vi "FSK.vi"() -> ()   [LabVIEW 2009]
uses:
  <vilib>/addons/Modulation/Analog/MT Downconvert Passband (Real).vi
  <vilib>/addons/Modulation/Analog/MT Upconvert Baseband (Real).vi
  <vilib>/addons/Modulation/Digital/General/MT Generate Bits (Galois, PN Order).vi
  <vilib>/Analysis/4window.llb/windowTd.ctl
  <vilib>/measure/maspectr.llb/FFT Power Spectrum for 1 Chan.vi
  Instance          11 16Saved   FSK-rev2 .vi
  <vilib>/Analysis/NI_AALPro.lvlib
  <vilib>/measure/NI_MAPro.lvlib
panel:
  in  "Tab Control":enum32{"Time Domain", "Frequency Domain"}(tab)
  out "Passband time domain signal":waveform(dbl)[](graph)=[{"t0"=timestamp(0 s since 1904-01-01), "dt"=4.166666666666667e-11, "Y"=array[25601 elements]}]
  out "Power Spectrum":cluster{"f0":dbl, "df":dbl, "spectrum":dbl[]}(graph)={"f0"=0.0, "df"=933815.8048324967, "spectrum"=array[12851 elements]}
  in  "symbol phase continuity":enum16{"continuous", "discontinuous"}(ring)=enum."discontinuous"
  out "df":dbl=933815.8048324967 format="%#_6p"
  in  "Frequency Deviation from Carrier (+/-)":dbl=500000000.0 format="%#_6p"
  in  "Random Sequence / 1010 Sequence":bool
  in  "modulation type 2":enum16{"FSK", "PSK", "QAM", "MSK", "PAM", "ASK"}(ring)
  in  "Delay per cycle (Seconds)":dbl=1.0 caption="Delay Time (s)"
  out "Symbol Period":dbl=8.333333333333334e-09
  out "Number of Bit Errors":i8
  out "Decoded Bits (16 shown at a time, scroll to view remainder)":i8[](array[numeric])=[0, 0, 0, 0, 1, 0, 0, 0, 0, 1, 1, 0, 0, 0, 1, 0, 1, 0, 0, 1, 1, 1, 1, 0, 1, 0, 0, 0, 1, 1, 1, 0, 0, 1, 0, 0, 1, 0, 1, 1, 0, 1, 1, 1, 0, 1, 1, 0, 0, 1, 1, 0, 1, 0, 1, 0, 1, 1, 1, 1, 1, 1, 0, 0, 0, 0, 0, 1, 0, 0, 0, 0, 1, 1, 0, 0, 0, 1, 0, 1, 0, 0, 1, 1, 1, 1, 0, 1, 0, 0, 0, 1, 1, 1, 0, 0, 1, 0, 0, 1, 0, 1, 1, 0, 1, 1, 1, 0, 1, 1, 0, 0, 1, 1, 0, 1, 0, 1, 0, 1, 1, 1, 1, 1, 1, 0]
  out "Signal Bandwidth":dbl=40000000.0 format="%#.6p"
  in  "Filter parameter (Rolloff Factor)":dbl=1.0 format="%.2f"
  in  "Carrier Frequency (Hz)":dbl=2000000000.0 min=-0.5 max=0.5 format="%#.6p"
  in  "modulation type":enum16{"FSK", "PSK", "QAM", "MSK", "PAM", "ASK"}(ring)=enum."ASK"
  in  "pulse shaping filter (none)":T1(ring)
  in  "filter length (symbols)":i32=8
  in  "Symbol Rate (Hz)":dbl=10000000.0 format="%#.6p"
  in  "Terminate Simulation":bool
  out "Bits (16 shown at a time, scroll to view remainder of stream)":i8[](array[numeric])=[0, 0, 0, 0, 1, 0, 0, 0, 0, 1, 1, 0, 0, 0, 1, 0, 1, 0, 0, 1, 1, 1, 1, 0, 1, 0, 0, 0, 1, 1, 1, 0, 0, 1, 0, 0, 1, 0, 1, 1, 0, 1, 1, 1, 0, 1, 1, 0, 0, 1, 1, 0, 1, 0, 1, 0, 1, 1, 1, 1, 1, 1, 0, 0, 0, 0, 0, 1, 0, 0, 0, 0, 1, 1, 0, 0, 0, 1, 0, 1, 0, 0, 1, 1, 1, 1, 0, 1, 0, 0, 0, 1, 1, 1, 0, 0, 1, 0, 0, 1, 0, 1, 1, 0, 1, 1, 1, 0, 1, 1, 0, 0, 1, 1, 0, 1, 0, 1, 0, 1, 1, 1, 1, 1, 1, 0, 0, 0]
  in  "PN sequence order (Valid range 6-15)":i32=6 min=5 max=31
  in  "Number of Bits to Generate":i32=128
  in  "Bit Sequence Generation Type  (Galois PN, Uniform Random)":bool
  # "Configuration"
  # "(delayed due to group delay of passband / pulse shaping / etc filters)"
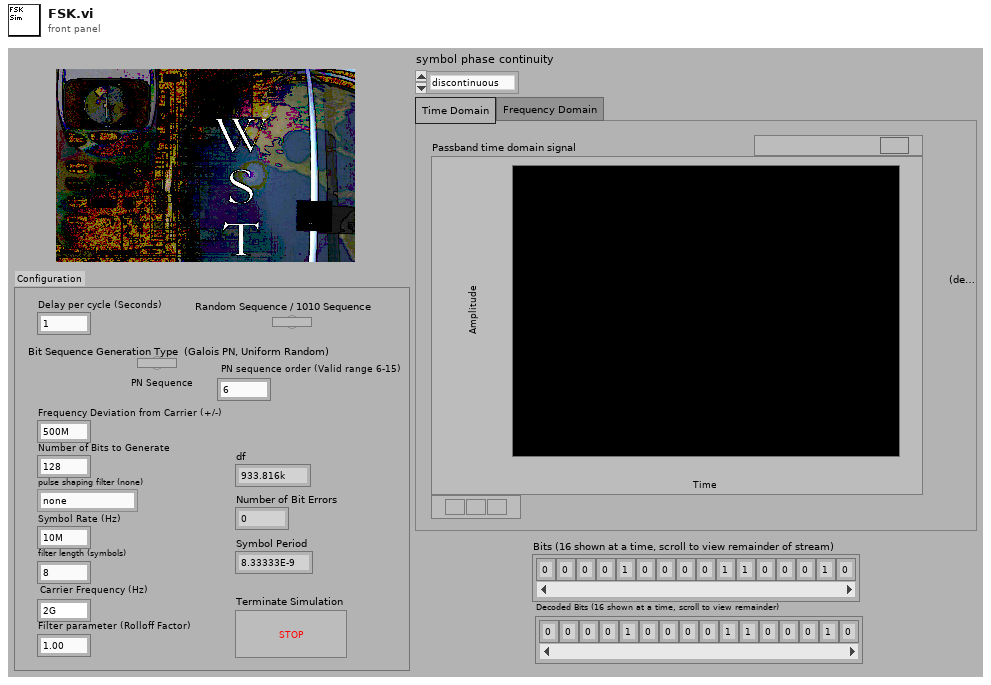
[diagram p1: front panel]
types:
  T1 = enum16{"none", "Raised Cosine", "Root Raised Cos"}
  T2 = enum16{"none", "Raised Cosine", "Root Raised Cos", "Gaussian"}
  T3 = cluster{"samples per symbol (16)":i32, "symbol map":dbl[], "symbol phase continuity":enum16{"continuous", "discontinuous"}}
  T4 = typedef "Complex Data Waveform.ctl" = cluster{"t0":dbl, "dt":dbl, "Y":cdb[]}
  T5 = typedef "NI_AALPro.lvlib/windowTd.ctl" = u32
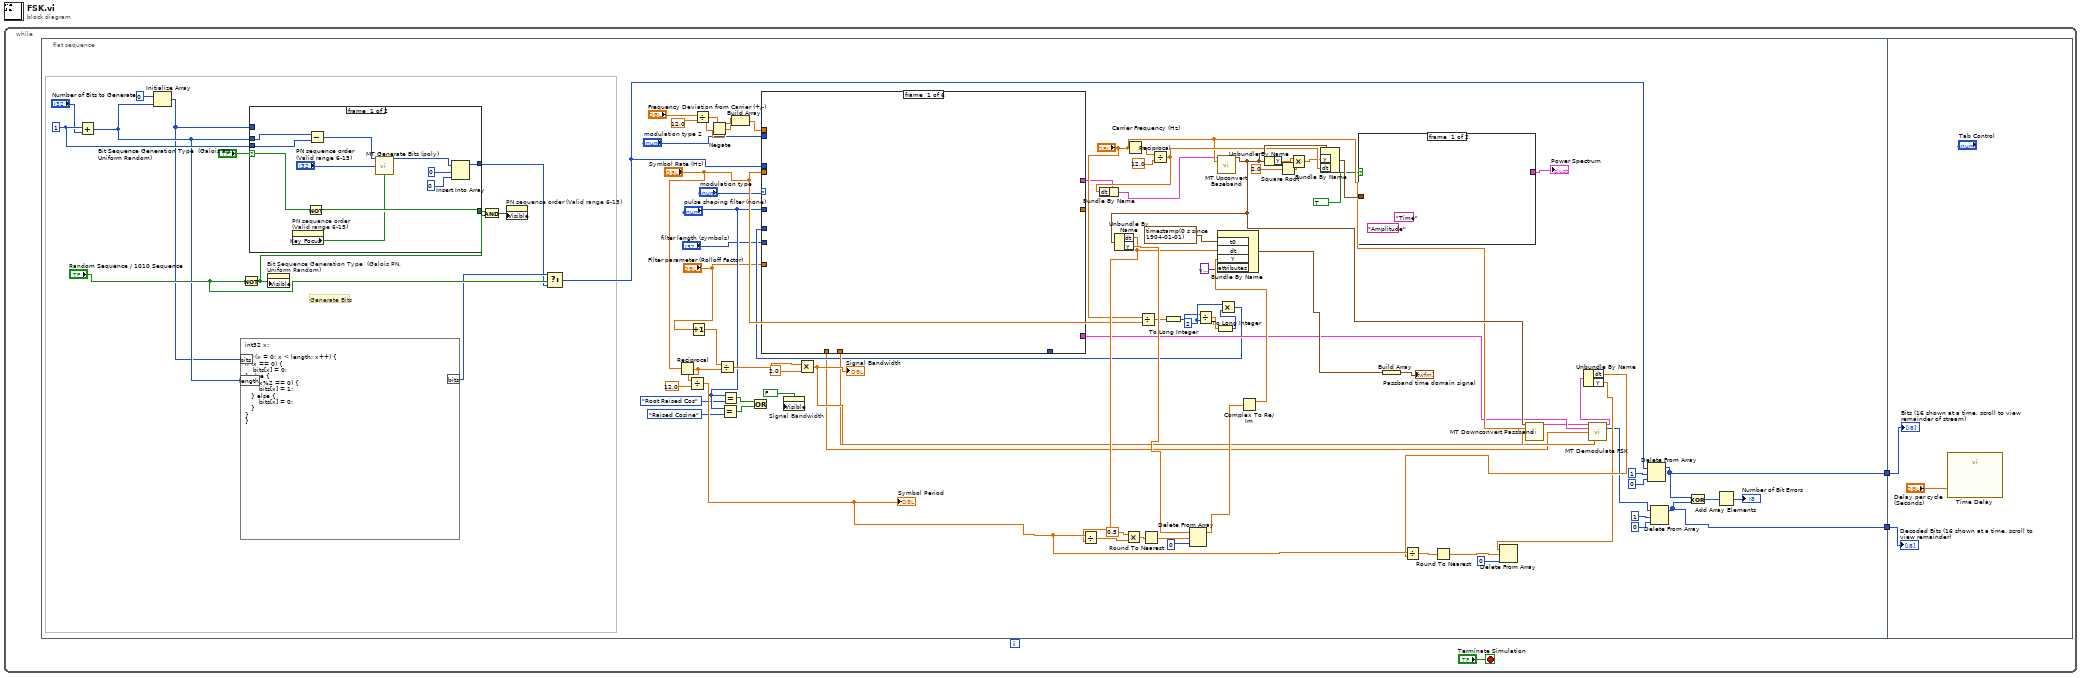
[diagram p0: block diagram]
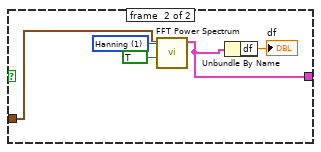
[diagram p2: hidden frame]
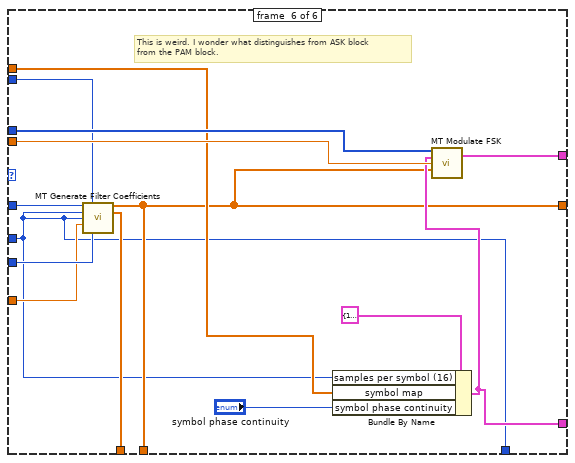
[diagram p7: hidden frame]
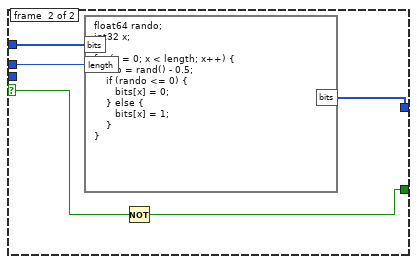
[diagram p8: hidden frame]
diagram:
  n1 = while {
    stop <- "Terminate Simulation" stop-if-true
    n2 = flat-sequence {
      tunnel: [w5] -> w2
      tunnel: [w4] -> w1
      tunnel: w2 -> [w128]
      tunnel: w1 -> [w127]
      frame #0 {
        w76 = 1 ("x")
        w21 = 2 ("y")
        # "Generate Bits"
        n3 = Add(x=w76, y="Number of Bits to Generate") -> (x+y=w50:i32)
        n4 = Initialize Array(i8 0, w50) -> (w49:i8[])
        n5 = formula code="int32 x;\n\nfor (x = 0; x < length; x++) {\nif (x == 0) {\n    bits[x] = 0;\n} else {\n   if (x%2 == 0) {\n       bits[x] = 1;\n   } else {\n       bits[x] = 0;\n   }\n}\n}"("bits"=w49, "length"=w50) -> ("bits"=w53:i8[])
        n6 = Not(x="Random Sequence / 1010 Sequence") -> (.not. x?=w57:bool)
        n7 = case shown="False" "Bit Sequence Generation Type  (Galois PN, Uniform Random)" {
          selector: "Bit Sequence Generation Type  (Galois PN, Uniform Random)" -> [w120 w123]
          tunnel: w50 -> [w113 w125]
          tunnel: [w114 w124] -> w52
          tunnel: w49 -> [_ w126]
          tunnel: [w119 w122] -> w55
          tunnel: w76 -> [w112 _]
          frame #0 {
            n8 = property on="PN sequence order (Valid range 6-15)" class="DigNum (strict)"() -> ("Key Focus"=w118:bool)  [unwired: 2 in, 2 out]
            n9 = Not(x=w120) -> (.not. x?=w119:bool)
            n10 = Subtract(x=w113, y=w112) -> (x-y=w117:i32)
            n11 = call-poly <vilib>:"MT Generate Bits (poly).vi"("total bits (128)"=w117, "PN sequence order (9)"="PN sequence order (Valid range 6-15)", "reset? (T)"=w118) -> ("output bit stream"=w115:i8[])  [unwired: 10 in, 2 out]
            n12 = Insert Into Array(array=w115, index=0, new element=i8 0 ("new element/subarray")) -> (w114:i8[])
          }
          frame #1 {
            n13 = formula code="float64 rando;\nint32 x;\n\nfor (x = 0; x < length; x++) {\nrando = rand() - 0.5;\n    if (rando <= 0) {\n       bits[x] = 0;\n    } else {\n       bits[x] = 1;\n    }\n}"("bits"=w126, "length"=w125) -> ("bits"=w124:i8[])
            n14 = Not(x=w123) -> (.not. x?=w122:bool)
          }
        }
        n15 = property on="Bit Sequence Generation Type  (Galois PN, Uniform Random)" class="Bool (strict)"("Visible"=w57) -> ()  [unwired: 2 in, 2 out]
        n16 = And(x=w55, y=w57) -> (x .and. y?=w56:bool)
        n17 = property on="PN sequence order (Valid range 6-15)" class="DigNum (strict)"("Visible"=w56) -> ()  [unwired: 2 in, 2 out]
        n18 = Select(t=w53, s="Random Sequence / 1010 Sequence", f=w52) -> (s? t:f=w85:i8[])
        n19 = Reciprocal(x="Symbol Rate (Hz)") -> (1/x=w30:dbl)
        n20 = Divide(x=w30, y=12.0) -> (x/y=w91:dbl)
        "Symbol Period" <- w91
        n21 = Increment(x="Filter parameter (Rolloff Factor)") -> (x+1=w11:dbl)
        n22 = Divide(x="Frequency Deviation from Carrier (+/-)", y=12.0) -> (x/y=w75:dbl)
        n23 = Negate(x=w75) -> (-x=w74:dbl)
        n24 = Divide(x=w11, y=w30) -> (x/y=w46:dbl)
        n25 = Equal?(x="pulse shaping filter (none)", y=T2."Raised Cosine") -> (x = y?=w13:bool)
        n26 = Equal?(x="pulse shaping filter (none)", y=T2."Root Raised Cos") -> (x = y?=w12:bool)
        n27 = Build Array(w74, w75) -> (w60:dbl[])
        n28 = Or(x=w12, y=w13) -> ()  [unwired: 1 out]
        n29 = property on="Signal Bandwidth" class="DigNum (strict)"("Visible"=FALSE) -> ()  [unwired: 2 in, 2 out]
        n30 = Multiply(x=w46, y=2.0) -> (x*y=w69:dbl)
        "Signal Bandwidth" <- w69
        n31 = Reciprocal(x="Carrier Frequency (Hz)") -> (1/x=w16:dbl)
        n32 = Divide(x="Carrier Frequency (Hz)", y="Symbol Rate (Hz)") -> (x/y=w19:dbl)
        n33 = Divide(x=w16, y=12.0) -> (x/y=w72:dbl)
        n34 = To Long Integer(number=w19) -> (32bit integer=w20:i32)
        n35 = Divide(x=w20, y=w21) -> (x/y=w22:dbl)
        n36 = To Long Integer(number=w22) -> (32bit integer=w23:i32)
        n37 = Multiply(x=w21, y=w23) -> (x*y=w26:i32)
        n38 = case shown="\"ASK\"" "modulation type" {
          tunnel: "Symbol Rate (Hz)" -> [_ _ _ _ _ w110]
          tunnel: "filter length (symbols)" -> [_ _ _ _ _ w109]
          tunnel: "pulse shaping filter (none)" -> [_ _ _ _ _ w108]
          tunnel: w85 -> [_ _ _ _ _ w107]
          tunnel: [_ _ _ _ _ w106] -> w61
          tunnel: "Filter parameter (Rolloff Factor)" -> [_ _ _ _ _ w105]
          tunnel: w26 -> [_ _ _ _ _ w97]
          tunnel: [_ _ _ _ _ w104] -> w25
          tunnel: "modulation type 2" -> [_ _ _ _ _ w103]
          tunnel: [_ _ _ _ _ w101] -> w58
          tunnel: [_ _ _ _ _ w98] -> w59
          tunnel: w60 -> [_ _ _ _ _ w100]
          tunnel: [_ _ _ _ _ w98] -> _
          tunnel: [_ _ _ _ _ w97] -> _
          frame #0 {
          }
          frame #1 {
          }
          frame #2 {
          }
          frame #3 {
          }
          frame #4 {
          }
          frame #5 {
            # "This is weird. I wonder what distinguishes from ASK block\nfrom the PAM block."
            n39 = call <vilib>:"MT Generate Filter Coefficients.vi"("pulse shaping filter (none)"=w108, "modulation type"=w103, "pulse shaping samples per symbol (16)"=w97, "matched samples per symbol (16)"=w97, "filter parameter"=w105, "filter length (symbols)"=w109) -> ("pulse shaping filter coefficients"=w98:dbl[], "matched filter coefficients"=w104:dbl[])  [unwired: 7 in, 1 out]
            n40 = Bundle By Name(cluster=T3 {"samples per symbol (16)"=16, "symbol map"=[], "symbol phase continuity"=enum."continuous"} ("FSK system parameters"), "samples per symbol (16)"=w97, "symbol map"=w100, "symbol phase continuity"="symbol phase continuity") -> (w101:T3)
            n41 = call <vilib>:"MT Modulate FSK.vi"("input bit stream"=w107, "FSK system parameters"=w101, "symbol rate (Hz)"=w110, "pulse shaping filter coefficients"=w98) -> ("output complex waveform"=w106:T4)  [unwired: 9 in, 2 out]
          }
        }
        n42 = Bundle By Name(cluster=w61, "dt"=w72) -> (w62:T4)
        n43 = call-poly <vilib>:"MT Upconvert Baseband.vi"("baseband waveform (complex)"=w62, "carrier frequency (Hz)"="Carrier Frequency (Hz)") -> ("passband waveform"=w87:waveform(dbl))  [unwired: 12 in, 1 out]
        n44 = Unbundle By Name(w87) -> ("dt"=w88:dbl, "Y"=w89:dbl[])
        n45 = Divide(x=w91, y=w88) -> (x/y=w77:dbl)
        n46 = Multiply(x=0.5, y=w77) -> (x*y=w79:dbl)
        n47 = Round To Nearest(number=w79) -> (nearest integer value=w90:dbl)
        n48 = Delete From Array(array=w89, length=w90, index=0) -> (array with subset deleted=w80:dbl[])  [unwired: 1 out]
        n49 = Complex To Re/Im(x + iy=w80) -> (x=w81:dbl[])  [unwired: 1 out]
        n50 = Bundle By Name("t0"=timestamp(0 s since 1904-01-01), "dt"=w88, "Y"=w81, "attributes"=variant) -> (w86:waveform(dbl))  [unwired: 1 in]
        n51 = Unbundle By Name(w87) -> ("Y"=w65:dbl[])
        n52 = Square Root(x=2.0) -> (sqrt(x)=w66:dbl)
        n53 = Multiply(x=w65, y=w66) -> (x*y=w68:dbl[])
        n54 = Bundle By Name(cluster=w87, "Y"=w68, "dt"=w72) -> (w82:waveform(dbl))
        n55 = case shown="True" TRUE {
          tunnel: [_ w93] -> w64
          tunnel: w82 -> [_ w92]
          frame #0 {
            (unwired) "Amplitude" ("X Scale.Name Label.Text")
            (unwired) "Time" ("X Scale.Name Label.Text")
          }
          frame #1 {
            w95 = T5 1 items=["Rectangle"=0, "Hanning"=1, "Hamming"=2, "Blackman-Harris"=3, "Exact Blackman"=4, "Blackman"=5, "Flat Top"=6, "4 Term B-Harris "=7, "7 Term B-Harris"=8, "Low Sidelobe"=9, "Blackman Nuttall"=11, "Triangle"=30, "Kaiser"=60, "Dolph-Chebyshev"=61, "Gaussian"=62] ("window")
            n56 = call-poly <vilib>:"FFT Power Spectrum.vi"("dB On (F)"=TRUE, "window"=w95, "time signal"=w92) -> ("power spectrum"=w93:cluster{"f0":dbl, "df":dbl, "magnitude":dbl[]})  [unwired: 5 in, 3 out]
            n57 = Unbundle By Name(w93) -> ("df"=→"df":dbl)
          }
        }
        "Power Spectrum" <- w64
        n58 = Build Array(w86) -> (→"Passband time domain signal":waveform(dbl)[])
        n59 = call-poly <vilib>:"MT Downconvert Passband.vi"("Waveform"=w87, "carrier frequency (Hz)"="Carrier Frequency (Hz)", "passband bandwidth (Hz)"=w69) -> ("downconverted waveform (complex baseband)"=w24:T4)  [unwired: 9 in, 3 out]
        n60 = call <vilib>:"MT Demodulate FSK.vi"("input complex waveform"=w24, "FSK system parameters"=w58, "matched filter coefficients"=w25, "pulse shaping filter coefficients"=w59) -> ("recovered complex waveform"=w29:T4, "output bit stream"=w37:i8[])  [unwired: 7 in, 3 out]
        n61 = Unbundle By Name(w29) -> ("dt"=w44:dbl, "Y"=w43:cdb[])
        n62 = Divide(x=w91, y=w44) -> (x/y=w40:dbl)
        n63 = Round To Nearest(number=w40) -> (nearest integer value=w41:dbl)
        n64 = Delete From Array(array=w43, length=w41, index=0) -> ()  [unwired: 2 out]
        n65 = Delete From Array(array=w85, length=1, index=0) -> (array with subset deleted=w5:i8[])  [unwired: 1 out]
        n66 = Delete From Array(array=w37, length=1, index=0) -> (array with subset deleted=w4:i8[])  [unwired: 1 out]
        n67 = Exclusive Or(1:w4, 2:w5) -> (0:w27:i8[])
        n68 = Add Array Elements(numeric array=w27) -> (sum=→"Number of Bit Errors":i8)
      }
      frame #1 {
        n69 = call "Time Delay"("Delay Time (s)"="Delay per cycle (Seconds)") -> ()  [unwired: 10 in, 1 out]
        "Decoded Bits (16 shown at a time, scroll to view remainder)" <- w127
        "Bits (16 shown at a time, scroll to view remainder of stream)" <- w128
      }
    }
  }
